vi "P-733 Format All Axes.vi"(7 "All Axis Array":string[](array[string])) -> (8 "All Axes String":string)   [LabVIEW 2016]
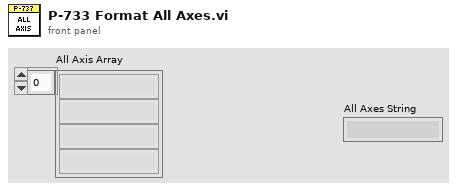
[diagram p1: front panel]
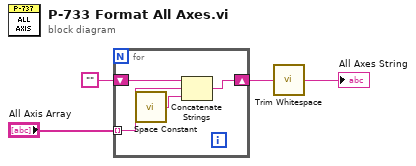
[diagram p0: block diagram]
diagram:
  n1 = for {
    tunnel: "All Axis Array" -> [w7] mode=indexing
    shift-right: [w5] -> w3
    shift-left: "" -> [w8]
    n2 = call <vilib>:"Space Constant.vi"() -> ("String"=w6:string)
    n3 = Concatenate Strings(w8, w7, w6) -> (w5:string)
  }
  n4 = call <vilib>:"Trim Whitespace.vi"("string"=w3) -> ("trimmed string"=→"All Axes String":string)  [unwired: 1 in]
